vi "ResetAndDefineConstants.vi"   [LabVIEW 2019]
doc: "This VI sets constants and resets the global variables."
uses:
  constants.vi
  outputs.vi
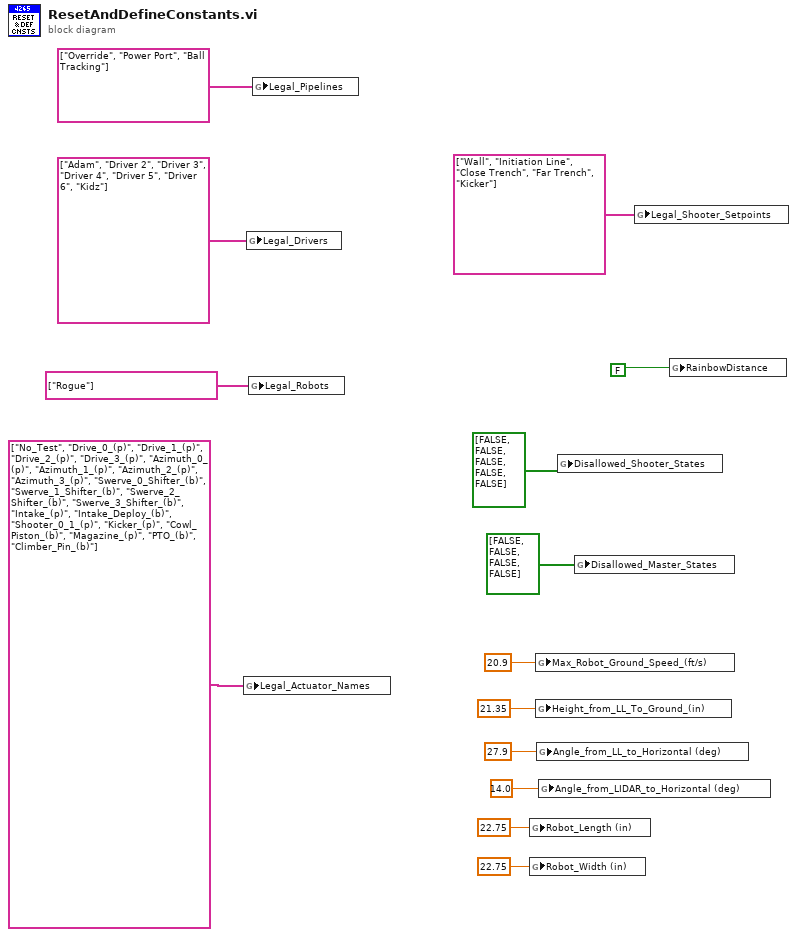
[diagram p0: block diagram]
diagram:
  n1 = global write "constants.vi" "Legal_Actuator_Names"(string[] ["No_Test", "Drive_0_(p)", "Drive_1_(p)", "Drive_2_(p)", "Drive_3_(p)", "Azimuth_0_(p)", "Azimuth_1_(p)", "Azimuth_2_(p)", "Azimuth_3_(p)", "Swerve_0_Shifter_(b)", "Swerve_1_Shifter_(b)", "Swerve_2_Shifter_(b)", "Swerve_3_Shifter_(b)", "Intake_(p)", "Intake_Deploy_(b)", "Shooter_0_1_(p)", "Kicker_(p)", "Cowl_Piston_(b)", "Magazine_(p)", "PTO_(b)", "Climber_Pin_(b)"] ("appended array")) -> ()
  n2 = global write "constants.vi" "Legal_Drivers"(string[] ["Adam", "Driver 2", "Driver 3", "Driver 4", "Driver 5", "Driver 6", "Kidz"] ("appended array")) -> ()
  n3 = global write "constants.vi" "Legal_Robots"(string[] ["Rogue"] ("Legal_Actuator_Names")) -> ()
  n4 = global write "constants.vi" "Legal_Pipelines"(string[] ["Override", "Power Port", "Ball Tracking"] ("appended array")) -> ()
  n5 = global write "constants.vi" "Robot_Length (in)"(22.75 ("Robot_Length (in)")) -> ()
  n6 = global write "constants.vi" "Robot_Width (in)"(22.75 ("Robot_Length (in)")) -> ()
  n7 = global write "constants.vi" "Max_Robot_Ground_Speed_(ft/s)"(20.9 ("Max_Robot_Ground_Speed_(ft/s)")) -> ()
  n8 = global write "constants.vi" "Height_from_LL_To_Ground_(in)"(21.35 ("Max_Robot_Ground_Speed_(ft/s)")) -> ()
  n9 = global write "constants.vi" "Angle_from_LL_to_Horizontal (deg)"(27.9 ("Max_Robot_Ground_Speed_(ft/s)")) -> ()
  n10 = global write "constants.vi" "Angle_from_LIDAR_to_Horizontal (deg)"(14.0 ("Angle_from_LIDAR_to_Horizontal (deg)")) -> ()
  n11 = global write "outputs.vi" "Disallowed_Shooter_States"(bool[] [FALSE, FALSE, FALSE, FALSE, FALSE] ("appended array")) -> ()
  n12 = global write "outputs.vi" "Disallowed_Master_States"(bool[] [FALSE, FALSE, FALSE, FALSE] ("appended array")) -> ()
  n13 = global write "constants.vi" "Legal_Shooter_Setpoints"(string[] ["Wall", "Initiation Line", "Close Trench", "Far Trench", "Kicker"] ("appended array")) -> ()
  n14 = global write "outputs.vi" "RainbowDistance"(FALSE) -> ()
